vi "Read Delay.vi"(8 "error in (no error)":errorcluster, 11 "Cheat in":refnum<class "Cheat.lvclass">) -> (0 "error out":errorcluster, 2 "Delay":dbl, 3 "Cheat out":refnum<class "Cheat.lvclass">)   [LabVIEW 2019, in "RT_Game.lvlib" / "Cheat.lvclass"]
uses:
  Cheat.lvclass
  Cheat.lvclass/Cheat.ctl
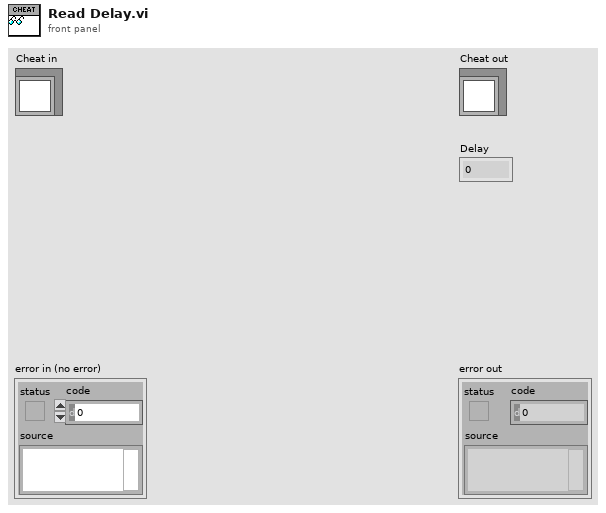
[diagram p1: front panel]
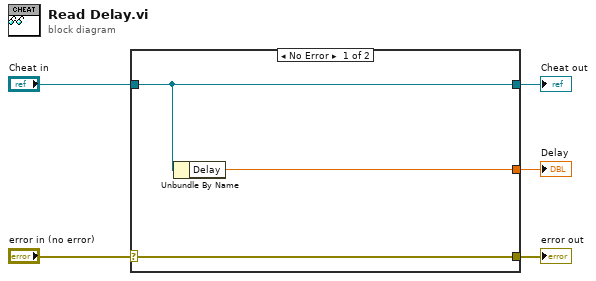
[diagram p0: block diagram]
diagram:
  n1 = case shown="No Error" "error in (no error)" {
    selector: "error in (no error)" -> [w8 w9]
    tunnel: [w8 w9] -> w4
    tunnel: [w7 w10] -> w2
    tunnel: "Cheat in" -> [w7 w10]
    tunnel: [w6 _] -> w1
    frame No Error {
      n2 = Unbundle By Name(w7) -> ("Delay"=w6:dbl)
    }
    frame Error {
    }
  }
  "error out" <- w4
  "Cheat out" <- w2
  "Delay" <- w1
